vi "Test Retrieve Record.vi"(8 "error in (no error)":errorcluster, 11 "Statement Refnum":T1) -> (0 "error out":errorcluster, 2 "Test Record":T2, 3 "Statement Refnum":T1)   [LabVIEW 2011]
uses:
  Test Record.ctl
  Summitek EXT/ODBC/SQL Controls/Statement Refnum.ctl
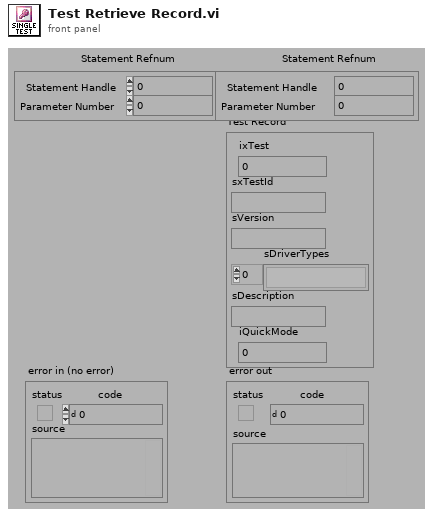
[diagram p1: front panel]
types:
  T1 = typedef "Statement Refnum.ctl" = cluster{"Statement Handle":i32, "Parameter Number":u16}
  T2 = typedef "Test Record.ctl" = cluster{"ixTest":i32, "sxTestId":string, "sVersion":string, "sDriverTypes":string[], "sDescription":string, "iQuickMode":i32}
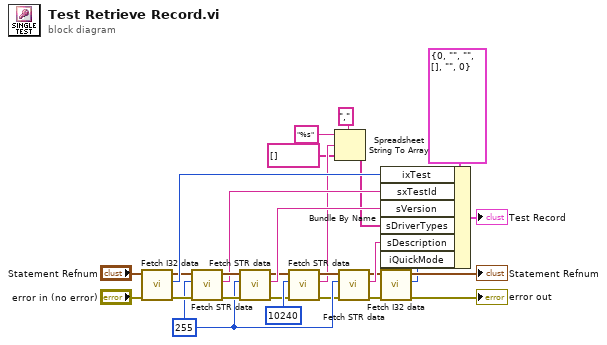
[diagram p0: block diagram]
diagram:
  w20 = 255 ("Buffer Size")
  n1 = call "Fetch I32 data.vi"("error in (no error)"="error in (no error)", "Statement Refnum"="Statement Refnum") -> ("error out"=w24:errorcluster, "Data"=w26:i32, "Statement Refnum"=w25:T1)  [unwired: 3 out]
  n2 = call "Fetch STR data.vi"("error in (no error)"=w24, "Buffer Size"=w20, "Statement Refnum"=w25) -> ("error out"=w22:errorcluster, "Data"=w19:string, "Statement Refnum"=w21:T1)  [unwired: 2 out]
  n3 = call "Fetch STR data.vi"("error in (no error)"=w22, "Buffer Size"=w20, "Statement Refnum"=w21) -> ("error out"=w2:errorcluster, "Data"=w18:string, "Statement Refnum"=w1:T1)  [unwired: 2 out]
  n4 = call "Fetch STR data.vi"("error in (no error)"=w2, "Buffer Size"=10240, "Statement Refnum"=w1) -> ("error out"=w15:errorcluster, "Data"=w12:string, "Statement Refnum"=w16:T1)  [unwired: 2 out]
  n5 = Spreadsheet String To Array(delimiter (Tab)=",", format string="%s", spreadsheet string=w12, array type (2D Dbl)=string[] []) -> (array=w9:string[])
  n6 = call "Fetch STR data.vi"("error in (no error)"=w15, "Buffer Size"=w20, "Statement Refnum"=w16) -> ("error out"=w5:errorcluster, "Data"=w17:string, "Statement Refnum"=w7:T1)  [unwired: 2 out]
  n7 = call "Fetch I32 data.vi"("error in (no error)"=w5, "Statement Refnum"=w7) -> ("error out"=→"error out":errorcluster, "Data"=w4:i32, "Statement Refnum"=→"Statement Refnum":T1)  [unwired: 3 out]
  n8 = Bundle By Name(cluster=T2 {"ixTest"=0, "sxTestId"="", "sVersion"="", "sDriverTypes"=[], "sDescription"="", "iQuickMode"=0} ("Test Information"), "ixTest"=w26, "sxTestId"=w19, "sVersion"=w18, "sDriverTypes"=w9, "sDescription"=w17, "iQuickMode"=w4) -> (→"Test Record":T2)
